vi "SubVI_EXA detector_trace.vi"(7 "Enable Auto Detector (T: Enable)":bool, 8 "error in (no error)":errorcluster, 9 "Trace Operation":u16(ring) items=["ClearWrite", "Average", "MaxHold", "MinHold"], 10 "Detector":u16(ring) items=["Average", "Peak", "Sample", "Nagative Peak"], 11 "VISA Refnum in":refnum<visa-resource-name>) -> (0 "error out":errorcluster, 3 "VISA resource name":refnum<visa-resource-name>)   [LabVIEW 2016]
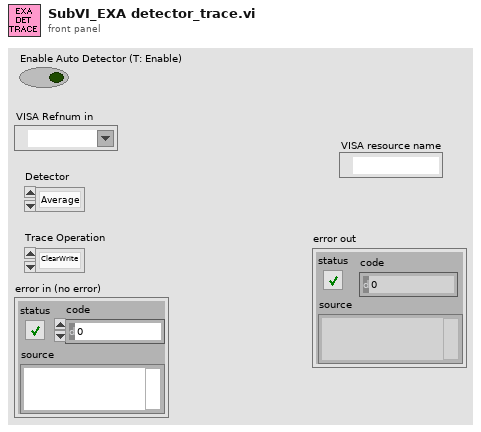
[diagram p1: front panel]
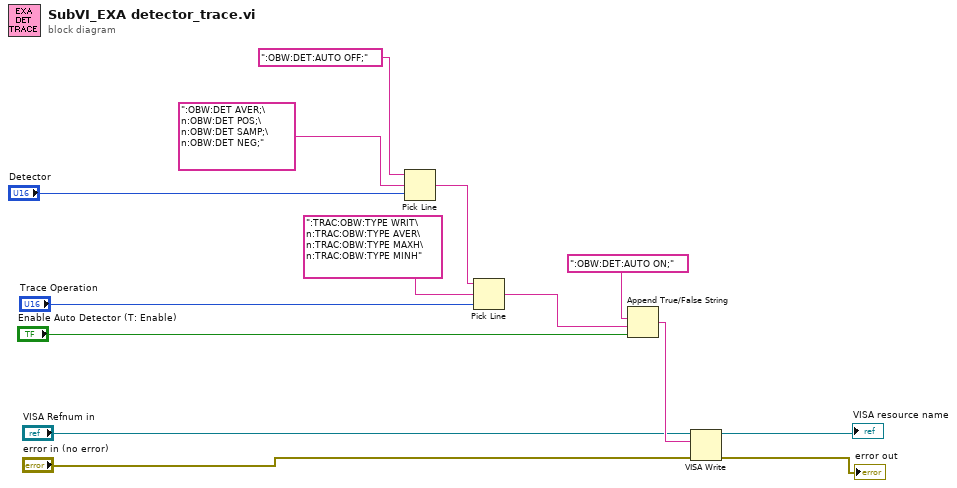
[diagram p0: block diagram]
diagram:
  n1 = Pick Line(string ("")=":OBW:DET:AUTO OFF;", multi-line string=":OBW:DET AVER;\n:OBW:DET POS;\n:OBW:DET SAMP;\n:OBW:DET NEG;" ("string (\"\")"), line index="Detector") -> (output string=w12:string)
  n2 = Pick Line(string ("")=w12, multi-line string=":TRAC:OBW:TYPE WRIT\n:TRAC:OBW:TYPE AVER\n:TRAC:OBW:TYPE MAXH\n:TRAC:OBW:TYPE MINH", line index="Trace Operation") -> (output string=w13:string)
  n3 = Append True/False String(1:"Enable Auto Detector (T: Enable)", 2:w13, 3:":OBW:DET:AUTO ON;" ("string (\"\")")) -> (0:w14:string)  [unwired: 1 in]
  n4 = VISA Write(VISA resource name="VISA Refnum in", write buffer=w14, error in (no error)="error in (no error)") -> (VISA resource name out=→"VISA resource name":refnum<visa-resource-name>, error out=→"error out":errorcluster)  [unwired: 1 out]
